vi "HandleInnerVITabbing.vi"(4 "Tab Backward To":refnum<vi>, 6 "Tab Forward To":refnum<vi>, 7 "Char":i16, 9 "Last Control":refnum<vi>, 10 "First Control":refnum<vi>, 11 "Shift":bool) -> (3 "Discard":bool)   [LabVIEW 2016]
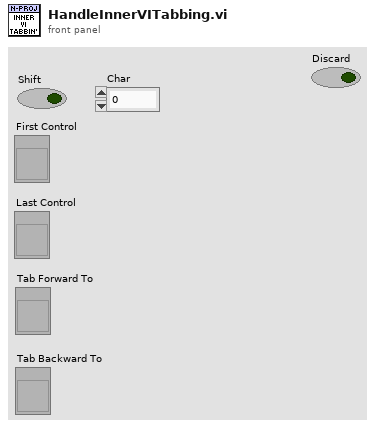
[diagram p1: front panel]
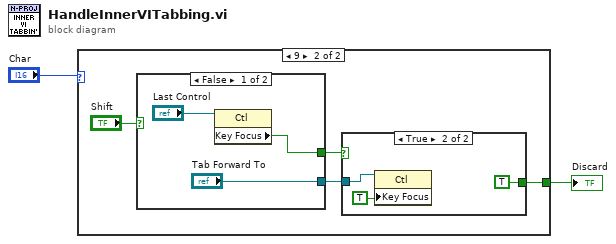
[diagram p0: block diagram]
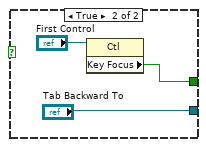
[diagram p3: hidden frame]
diagram:
  n1 = case shown="9" "Char" {
    tunnel: [_ w4] -> w2
    frame Default {
    }
    frame 9 {
      n2 = case shown="False" "Shift" {
        tunnel: [w9 w12] -> w5
        tunnel: ["Tab Forward To" "Tab Backward To"] -> w6
        frame False {
          n3 = property on="Property Node" class="Ctl"(reference="Last Control") -> ("Key Focus"=w9:bool)  [unwired: 1 in, 2 out]
        }
        frame True {
          n4 = property on="Property Node" class="Ctl"(reference="First Control") -> ("Key Focus"=w12:bool)  [unwired: 1 in, 2 out]
        }
      }
      n5 = case shown="True" w5 {
        tunnel: w6 -> [_ w15]
        tunnel: [_ TRUE] -> w4
        frame False {
        }
        frame True {
          n6 = property on="Property Node" class="Ctl"(reference=w15, "Key Focus"=TRUE) -> ()  [unwired: 1 in, 2 out]
        }
      }
    }
  }
  "Discard" <- w2
